vi "setPolarity.vi"(0 "Controller in":refnum<class "_Controller.lvclass">, 2 "polarity_items (in)":T2[](array[typedef]), 3 "axis (in)":T1, 5 "error in (no error)":errorcluster) -> (14 "Controller out":refnum<class "_Controller.lvclass">, 17 "success?":bool, 18 "response":string, 19 "error out":errorcluster)   [LabVIEW 2013, in "classes.lvlib" / "_Controller.lvclass"]
doc: "Sets the Polarity Value(s) for a given axis. For single axis applications, the axis input need not be used.\n\nThis VI takes as input an array of polarity \"items\". Each item consists of an item name and an item value. The item name is selectable from list of available polarity definitions that may or may not be applicable to the referenced controller. Please refer to the supporting documenation for the referenced controller if there is any confusion about whether a given polarity item is supported.\n\nProduced By:\n\n<B>Kod Integrations, LLC</B>\n4835 Marianne Drive\nMount Airy, MD 21771\nhttp://www.kodintegrations.com\nemail: info@kodintegrations.com\nphone: (240) 687-1288"
uses:
  _Controller.lvclass
  common/controls/polarity_item.ctl
  common/controls/polarity.ctl
  common/controls/axis.ctl
  libraries/common.lvlib
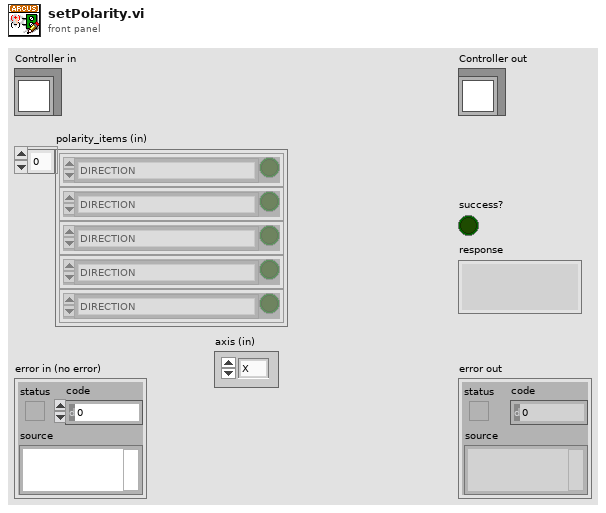
[diagram p1: front panel]
types:
  T1 = typedef "common.lvlib/axis.ctl" = enum16{"X", "Y", "Z", "U"}
  T2 = typedef "common.lvlib/polarity_item.ctl" = cluster{"item":T3, "status":bool}
  T3 = typedef "common.lvlib/polarity.ctl" = enum16{"DIRECTION", "LIMIT", "HOME", "DIG_OUT", "DIG_IN", "ENABLE_OUT", "JUMP_ERR", "LATCH", "Z-CHAN_INDEX", "ENCODER_DECODING:1X", "ENCODER_DECODING:2X", "ENCODER_DECODING:4X", "ALARM", "STANDALONE_ERR", "-", "<reserved/nc>"}
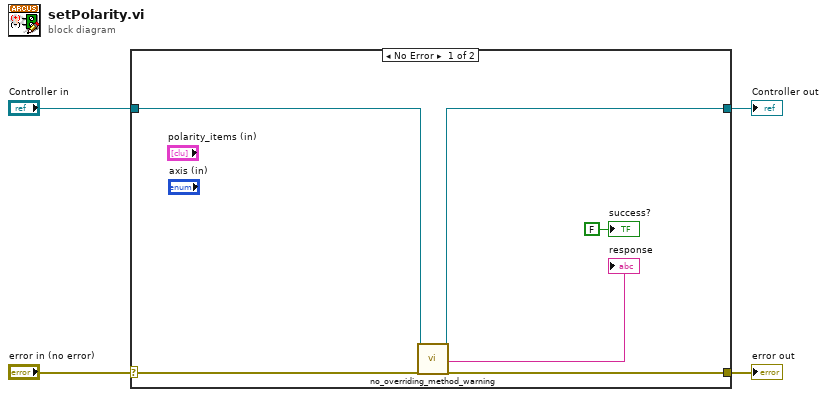
[diagram p0: block diagram]
diagram:
  n1 = case shown="No Error" "error in (no error)" {
    selector: "error in (no error)" -> [w10 w12]
    tunnel: [w9 w12] -> w3
    tunnel: [w7 w11] -> w1
    tunnel: "Controller in" -> [w8 w11]
    frame No Error {
      n2 = call "no_overriding_method_warning.vi"("Controller (in)"=w8, "error in (no error)"=w10) -> ("Controller (out)"=w7:refnum<class "_Controller.lvclass">, "msg"=→"response":string, "error out"=w9:errorcluster)  [unwired: 15 in]
      "success?" <- FALSE ("success?")
    }
    frame Error {
    }
  }
  "error out" <- w3
  "Controller out" <- w1
